vi "IV read SN.vi"(8 "error in (no error)":errorcluster, 11 "sntext":string) -> (0 "error out":errorcluster, 2 "return type":i32, 3 "sntext out":string)   [LabVIEW 2020, in "IVIUM_remdriver.lvlib"]
uses:
  IVIUM_remdriver.lvlib
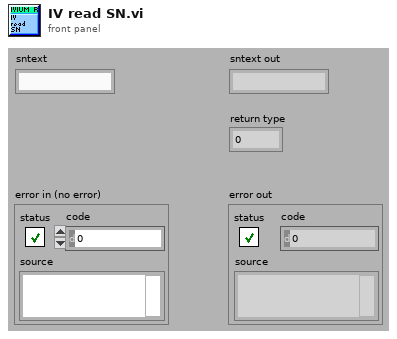
[diagram p1: front panel]
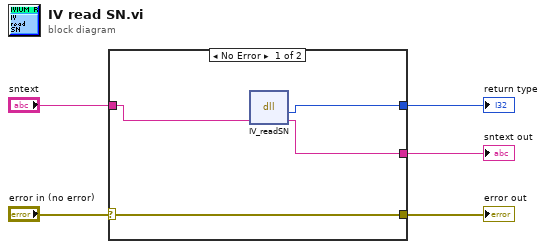
[diagram p0: block diagram]
diagram:
  n1 = case shown="No Error" "error in (no error)" {
    selector: "error in (no error)" -> [w9 w11]
    tunnel: [w9 w11] -> w4
    tunnel: [w8 _] -> w3
    tunnel: "sntext" -> [w7 w10]
    tunnel: [w6 w10] -> w1
    frame No Error {
      n2 = dll-call lib="IVIUM_remdriver" fn="IV_readSN"("sntext"=w7) -> ("return type"=w8:i32, "sntext"=w6:string)  [unwired: 3 in, 2 out]
    }
    frame Error {
    }
  }
  "return type" <- w3
  "sntext out" <- w1
  "error out" <- w4
